vi "Dequeue Message.vi"(8 "error in (no error)":errorcluster, 11 "Message Queue":refnum<queue>) -> (0 "error out":errorcluster, 1 "Message Data":variant, 2 "Message":string, 3 "dup Message Queue":refnum<queue>)   [LabVIEW 2013, in "Message Queue.lvlib"]
doc: "This VI pulls messages off the Message Queue. It has special error handling to account for an error occurring on the last iteration of the Message Handling Loop.\n\nNo Error - normal Dequeue Element operation.\nError - check if it is an error code we wish to ignore. If so, clear the error and perform a normal Dequeue Element. If not, output the error, and put a 'Stop' message on the Message Queue."
uses:
  Message Queue.lvlib
  Message Cluster.ctl
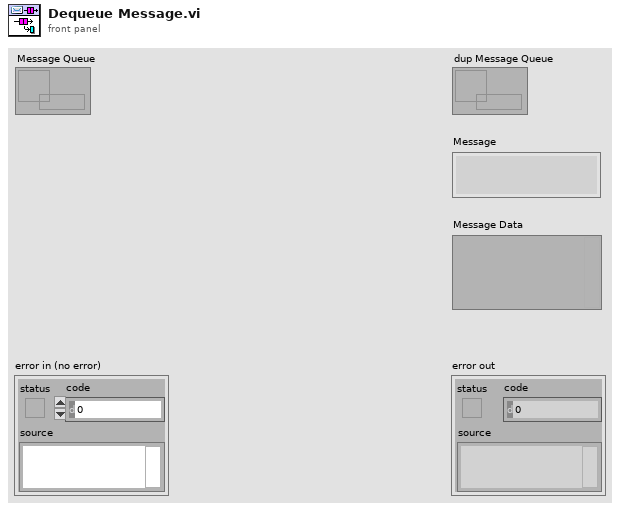
[diagram p1: front panel]
types:
  T1 = typedef "Message Queue.lvlib/Message Cluster.ctl" = cluster{"Message":string, "Message Data":variant}
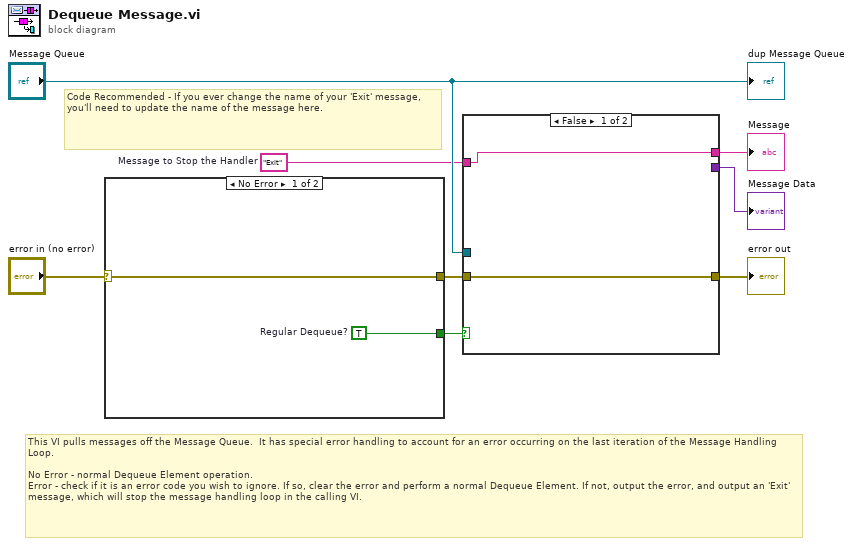
[diagram p0: block diagram]
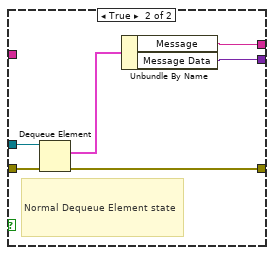
[diagram p2: hidden frame]
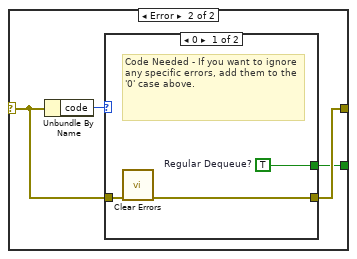
[diagram p3: hidden frame]
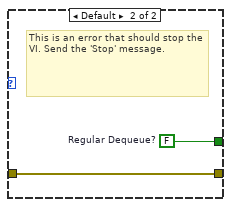
[diagram p4: hidden frame]
diagram:
  w1 = "Exit"  # Message to Stop the Handler
  # "Code Recommended - If you ever change the name of your 'Exit' message, you'll need to update the name of the message here."
  # "This VI pulls messages off the Message Queue.  It has special error handling to account for an error occurring on the last iteration of the Message Handling Loop.\n\nNo Error - normal Dequeue Element operation.\nError - check if it is an error code you wish to ignore. If so, clear the error and perform a normal Dequeue Element. If not, output the error, and output an 'Exit' message, which will stop the message handling loop in the calling VI."
  n1 = case shown="No Error" "error in (no error)" {
    selector: "error in (no error)" -> [w10 w13]
    tunnel: [w10 w12] -> w6
    tunnel: [w9 w11] -> w5
    frame No Error {
      w9 = TRUE  # Regular Dequeue?
    }
    frame Error {
      n2 = Unbundle By Name(w13) -> ("code"=w14:i32)
      n3 = case shown="0" w14 {
        tunnel: [w17 w19] -> w12
        tunnel: w13 -> [w16 w19]
        tunnel: [w15 w18] -> w11
        frame 0 {
          w15 = TRUE  # Regular Dequeue?
          # "Code Needed - If you want to ignore any specific errors, add them to the '0' case above."
          n4 = call <vilib>:"Clear Errors.vi"("error in (no error)"=w16) -> ("error out"=w17:errorcluster)  [unwired: 6 in]
        }
        frame Default {
          w18 = FALSE  # Regular Dequeue?
          # "This is an error that should stop the VI. Send the 'Stop' message."
        }
      }
    }
  }
  n5 = case shown="False" w5 {
    tunnel: [w21 w27] -> w7
    tunnel: w6 -> [w21 w26]
    tunnel: "Message Queue" -> [_ w25]
    tunnel: [w20 w23] -> w3
    tunnel: [_ w22] -> w2
    tunnel: w1 -> [w20 _]
    frame False {
    }
    frame True {
      # "Normal Dequeue Element state"
      n6 = Dequeue Element(queue=w25, error in (no error)=w26) -> (element=w24:T1, error out=w27:errorcluster)  [unwired: 1 in, 2 out]
      n7 = Unbundle By Name(w24) -> ("Message"=w23:string, "Message Data"=w22:variant)
    }
  }
  "error out" <- w7
  "Message" <- w3
  "Message Data" <- w2
  "dup Message Queue" <- "Message Queue"
